vi "Transfer Group.Get Direction.vi"(11 "Transfer Group in":refnum<class "Transfer Group.lvclass">) -> (2 "Direction":T1, 3 "Transfer Group out":refnum<class "Transfer Group.lvclass">)   [LabVIEW 2017, in "DSF Core.lvlib" / "Transfer Group.lvclass"]
uses:
  Transfer Group.lvclass
  DSF Configuration API/Public/Controls/DSF Direction.ctl
  Transfer Group.lvclass/Transfer Group.ctl
  DSF Configuration.lvlib
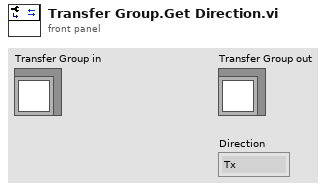
[diagram p1: front panel]
types:
  T1 = typedef "DSF Configuration.lvlib/DSF Direction.ctl" = enum8{"Tx", "Rx"}
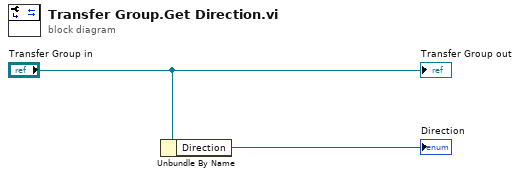
[diagram p0: block diagram]
diagram:
  n1 = Unbundle By Name("Transfer Group in") -> ("Direction"=→"Direction":T1)
  "Transfer Group out" <- "Transfer Group in"
